vi "Generate Patch Seq Img Core-retd.vi"(0 "tdms file ref":refnum<k34>, 1 "Channel to process":enum16{"Red", "Green"}(ring), 5 "All header parameters":T1={"Imaging Protocol"=enum."AOL Z-Stack", "Number of POI"=0, "Number of Miniscans"=0, "Number of Trials"=0, "Number of Cycles "=0, "# Averaged Frames"=0, "Laser power (%)"=0, "Pockels"=0.0, "Acquisition Length (sec)"=0.0, "Fill time (us)"=0.0, "POI Dwell time (us)"=0.0, "Miniscan Dwell time per pixel (us)"=0.0, "PMT 1"=0.0, "PMT 2"=0.0, "Back Apperture"=0.0, "Zoom"=0.0, "Frame Size"=200, "Center Frequency"=0.0, "Field of View"=0.0, "DwellTime (us)"=0.0, "Wavelength (nm)"=0.0, "AOL Z"=0.0, "AOL Mode"=enum."Raster", "GridXY"=0.0, "GridZ"=0.0, "TriggerDelay (sec)"=0.0, "Number of Pixels in Miniscan"=0, "Experiment folder path"=path "", "X centre"=0.0, "Y centre"=0.0, "Angle (degrees)"=0.0, "Plane Mode"=0, "Software version"=0.0, "Objective"="Olympus  20X", "MotorZ Calibration"=0, "Pockels Calibration"=0, "Threshold"=[], "Video length (sec)"=0.0, "Frame rate (fps)"=0, "Rectangle ROI length (pixels)"=0, "Rectangle ROI height (pixels)"=0} {"Pockels" format="%#.6g"; "Software version" format="%#.6g"; "Plane Mode" items=["XY Plane", "XZ Plane", "YZ Plane", "arbitraryplane"]; "Angle (degrees)" format="%#.6g"; "Frame Size" items=["100X100"=100, "128X128"=128, "200X200"=200, "256X256"=256, "512X512"=512, "1024x1024"=1024, "2048x2048"=2048]; "Back Apperture" format="%#.6g"; "PMT 2" format="%#.6g"; "PMT 1" format="%#.6g"; "Miniscan Dwell time per pixel (us)" format="%#.6g"; "Zoom" format="%#.6g"; "POI Dwell time (us)" format="%#.6g"; "Acquisition Length (sec)" format="%#.6g"; "Fill time (us)" format="%#.6g"}, 7 "TDMS file path & name":path=path "C:/Users/Theo/Desktop/Datasets/140401_17_44_08-rig 3 debugging/Functional imaging TDMS data files/001.tdms", 9 "Patch Image Folder":path[](array[path]), 11 "error in (no error)":errorcluster, 13 "TIFF file handles":i32[](array[numeric]), 14 "Trial Number":i32) -> (4 "tdms file out":refnum<k34>, 15 "error out":errorcluster)   [LabVIEW 2020]
uses:
  User Interface/Visualisation/Functional Imaging Viewer/SubVIs/Experiment header interface/Typedefs/Header parameters cluster-ALL-retd.ctl
  Typedefs/Imaging Protocols enum.ctl
  Typedefs/Frame Size.ctl
  Typedefs/AOL modes.ctl
  Typedefs/Plane Mode.ctl
  Typedefs/Objective selector control enum.ctl
  Typedefs/Channel Selector.ctl
  Globals/gl_funct TIFF export globals.vi
  <vilib>/vision/NI_Vision_Development_Module.lvlib
panel:
  out "Loop time (ms)":u32
  # "Re-entrant"
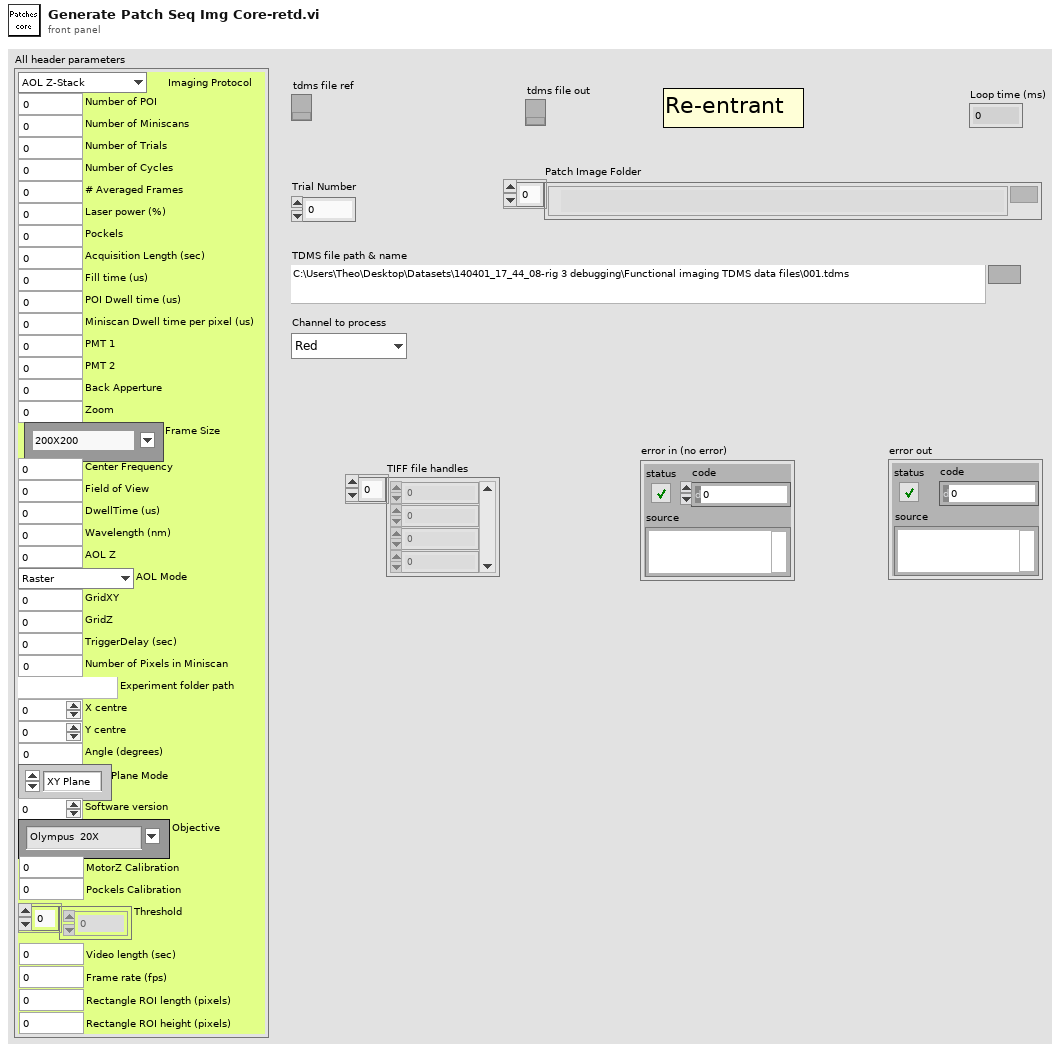
[diagram p1: front panel]
types:
  T1 = typedef "Header parameters cluster-ALL-retd.ctl" = cluster{"Imaging Protocol":T2, "Number of POI":u16, "Number of Miniscans":u16, "Number of Trials":u16, "Number of Cycles ":u64, "# Averaged Frames":u16, "Laser power (%)":u8, "Pockels":dbl, "Acquisition Length (sec)":dbl, "Fill time (us)":dbl, "POI Dwell time (us)":dbl, "Miniscan Dwell time per pixel (us)":dbl, "PMT 1":dbl, "PMT 2":dbl, "Back Apperture":dbl, "Zoom":dbl, "Frame Size":T3, "Center Frequency":dbl, "Field of View":dbl, "DwellTime (us)":dbl, "Wavelength (nm)":dbl, "AOL Z":dbl, "AOL Mode":T4, "GridXY":dbl, "GridZ":dbl, "TriggerDelay (sec)":dbl, "Number of Pixels in Miniscan":u16, "Experiment folder path":path, "X centre":dbl, "Y centre":dbl, "Angle (degrees)":dbl, "Plane Mode":T5, "Software version":dbl, "Objective":T6, "MotorZ Calibration":u32, "Pockels Calibration":u32, "Threshold":u16[], "Video length (sec)":dbl, "Frame rate (fps)":u8, "Rectangle ROI length (pixels)":u16, "Rectangle ROI height (pixels)":u16}
  T2 = typedef "Imaging Protocols enum.ctl" = enum16{"AOL Z-Stack", "Motor Z Stack", "Functional Acquisition", "Single Plane Acquisition", "Volume Acquisition", "Live Imaging", "Live Plane Imaging", "Live Volume Imaging"}
  T3 = typedef "Frame Size.ctl" = u16
  T4 = typedef "AOL modes.ctl" = enum16{"Raster", "Structural", "Pointing", "Mini Scan", "Alignment"}
  T5 = typedef "Plane Mode.ctl" = u16
  T6 = typedef "Objective selector control enum.ctl" = string
  T7 = typedef "Funct TIFF exporter ctrl refs.ctl" = cluster{"This VI":refnum<vi>, "Current Experiment":refnum<vi>, "Imaging protocol":refnum<vi>, "Predominant ROI type":refnum<vi>, "Patches in Experiment":refnum<vi>, "Folder Path":refnum<vi>, "Export":refnum<vi>, "Trial number":refnum<vi>, "Output TIFF type":refnum<vi>}
  T8 = typedef "Exported TIFF type.ctl" = enum16{"One multi-page TIFF file for each rectangle", "Individual TIFF files"}
  T9 = typedef "Channel Selector.ctl" = enum16{"Red Channel", "Green Channel", "Blended"}
  T10 = cluster{"Number of cycles":i32, "number of planes":i32, "number of miniscans in a Plane":i32, "number of pixels in a miniscan":i32}
  T11 = typedef "Image Type" = u32
  T12 = typedef "IMAQ Image.ctl" = refnum<image>
  T13 = typedef "IMAQ AVI2 Refnum.ctl" = refnum<k20>
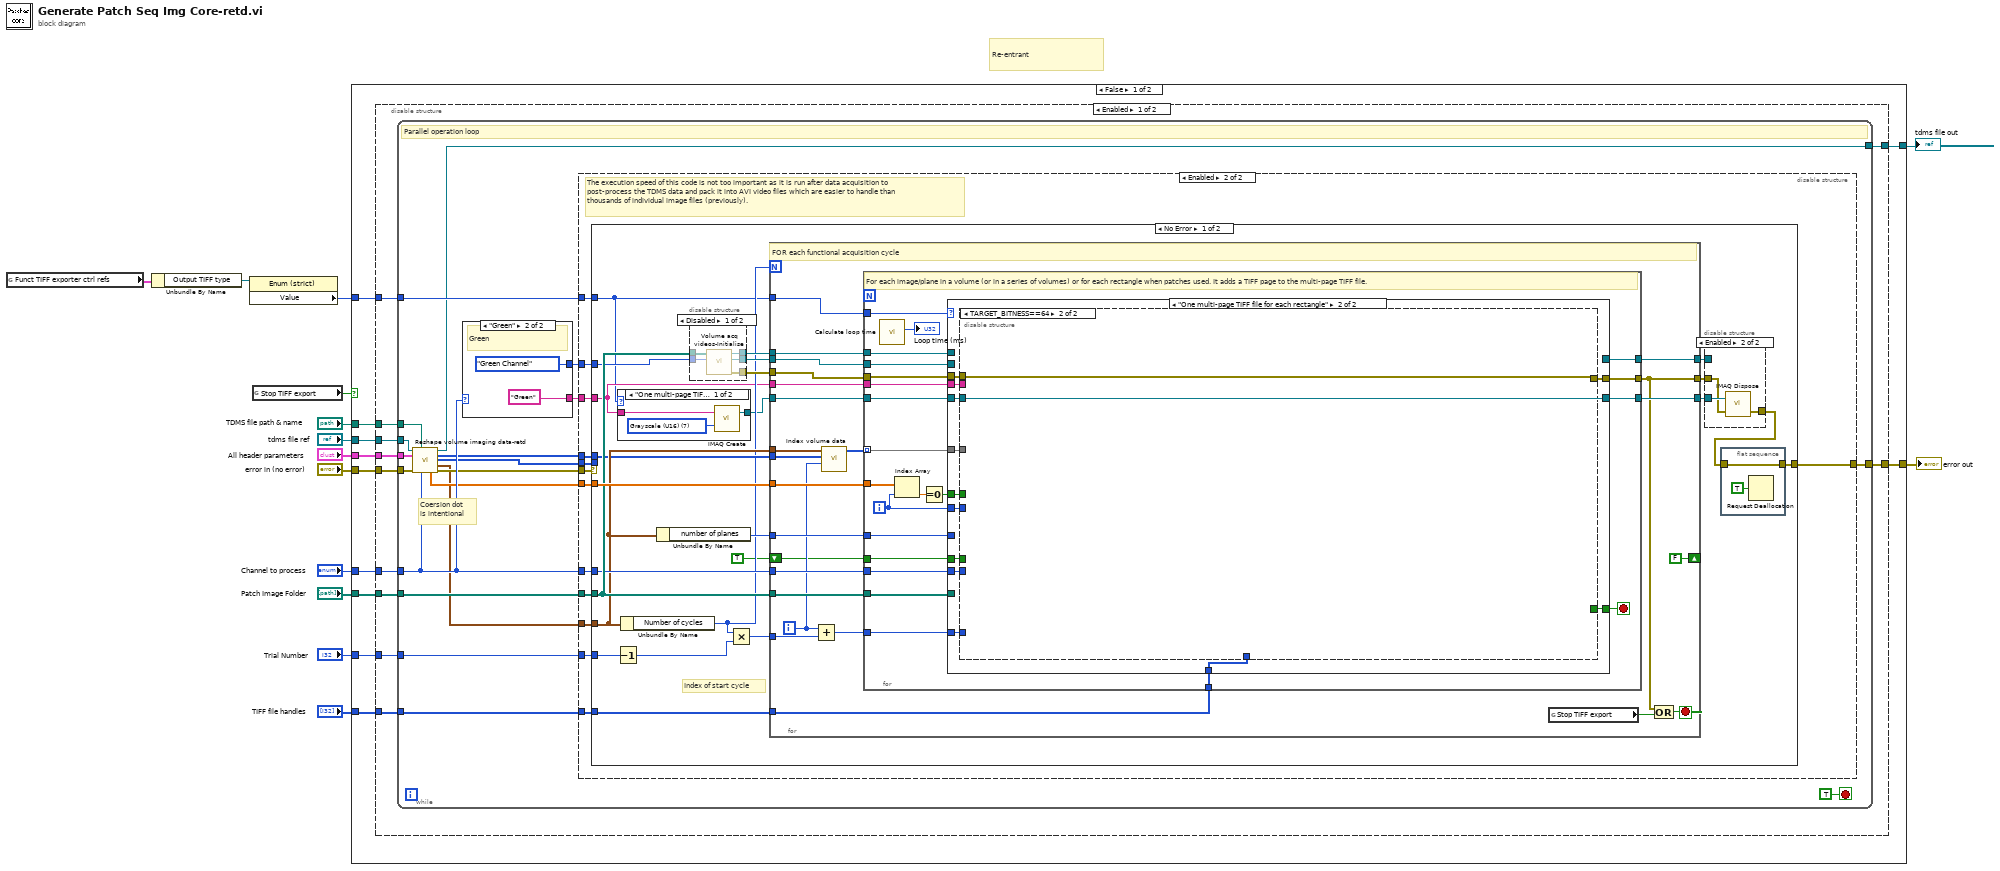
[diagram p0: block diagram]
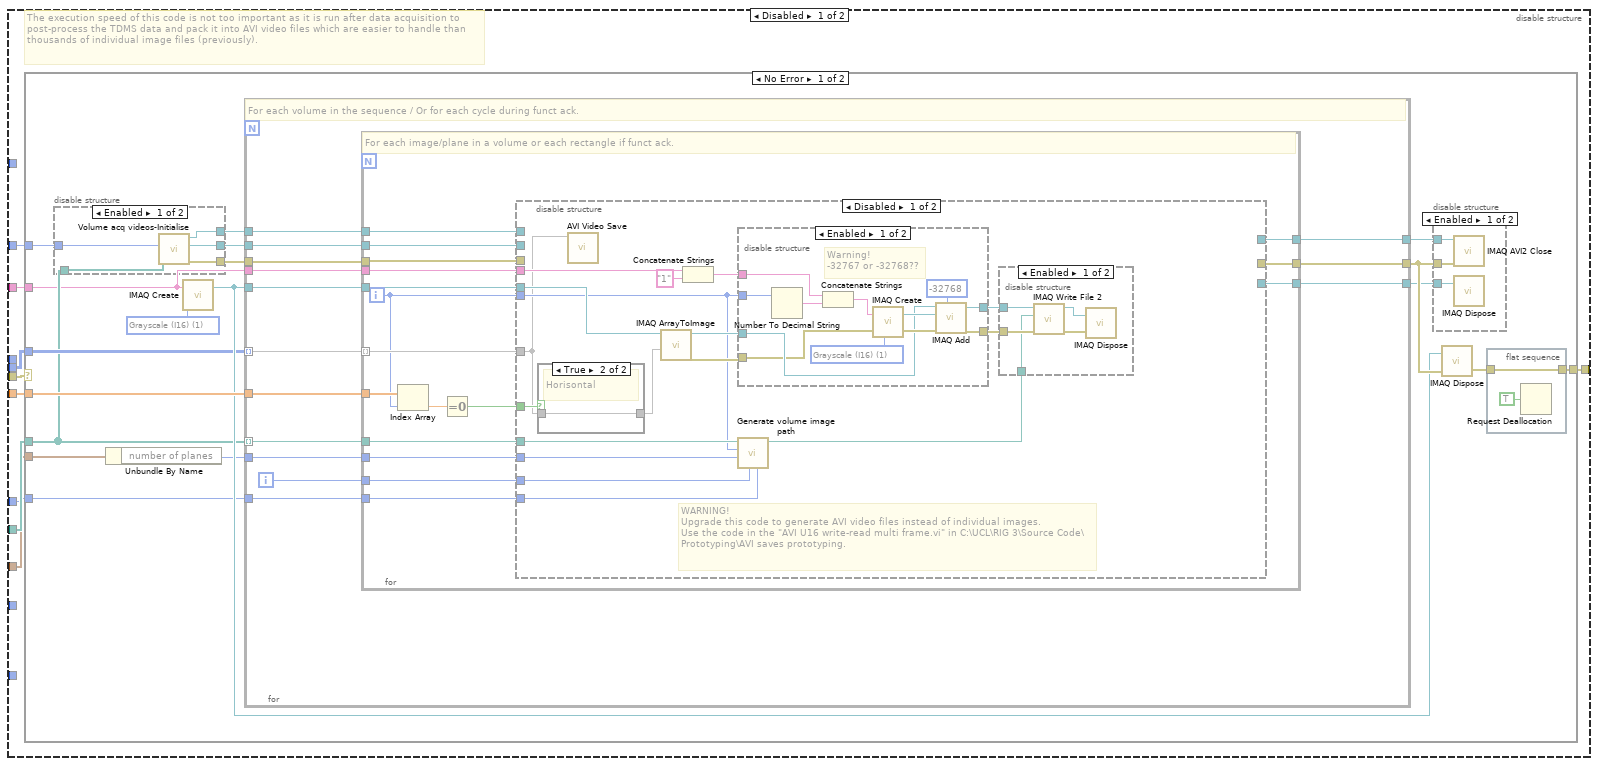
[diagram p2: hidden frame]
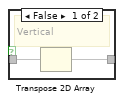
[diagram p5: hidden frame]
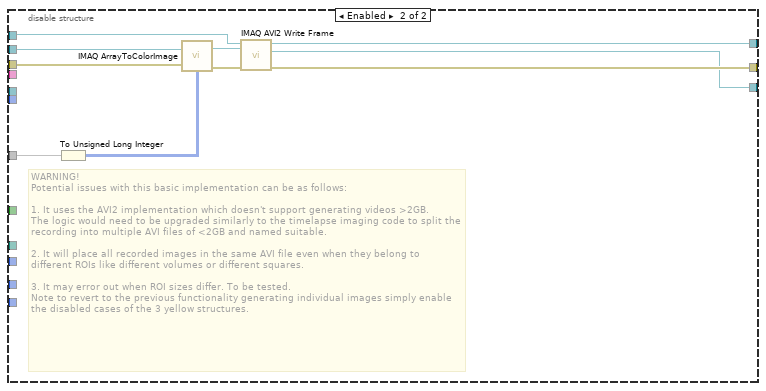
[diagram p8: hidden frame]
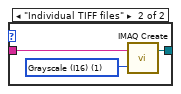
[diagram p10: hidden frame]
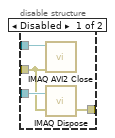
[diagram p12: hidden frame]
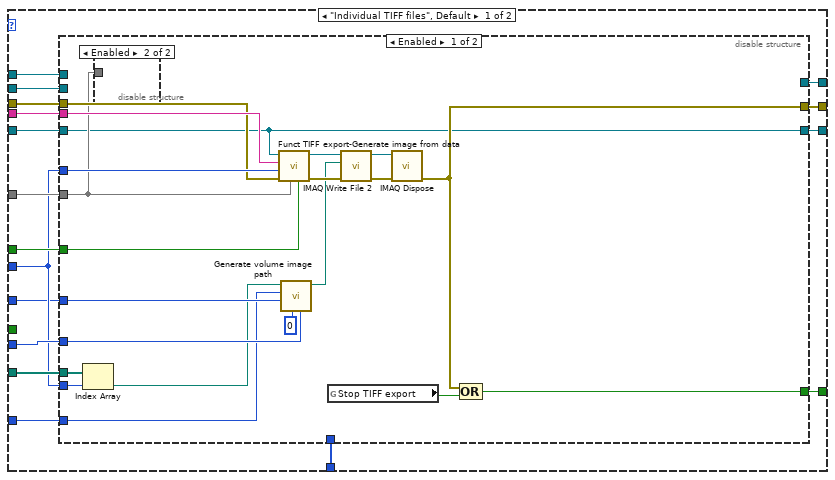
[diagram p13: hidden frame]
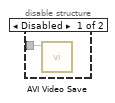
[diagram p14: hidden frame]
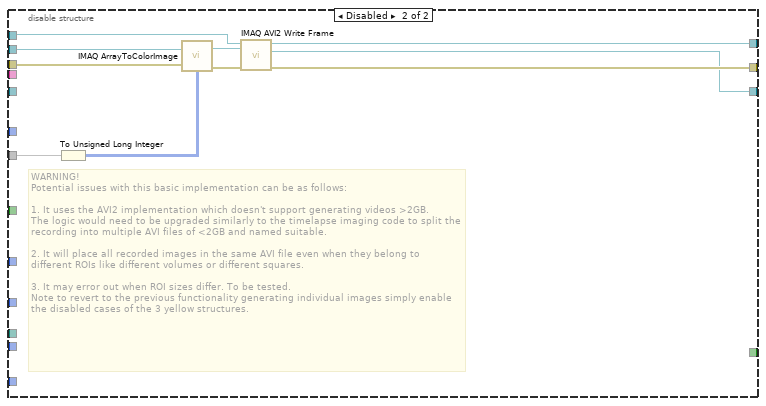
[diagram p15: hidden frame]
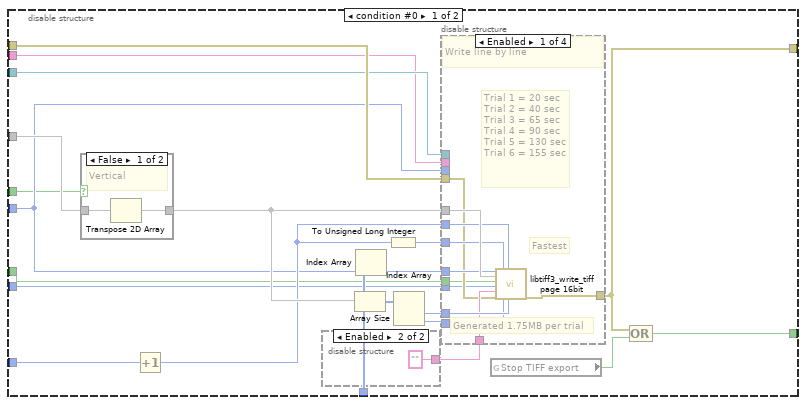
[diagram p16: hidden frame]
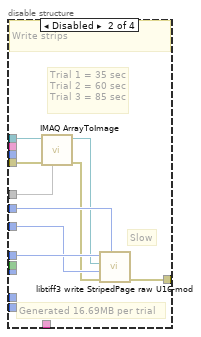
[diagram p17: hidden frame]
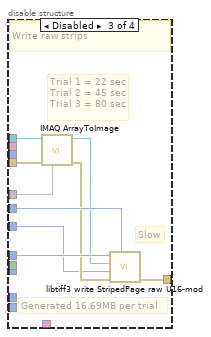
[diagram p18: hidden frame]
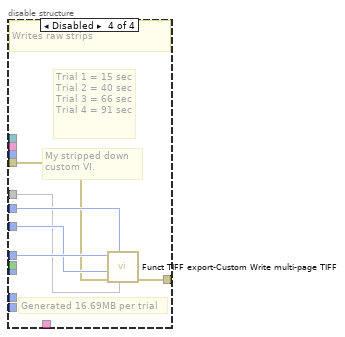
[diagram p19: hidden frame]
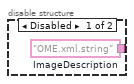
[diagram p20: hidden frame]
diagram:
  # "Re-entrant"
  n1 = global read "gl_funct TIFF export globals.vi" "Funct TIFF exporter ctrl refs"() -> (w6:T7)
  n2 = Unbundle By Name(w6) -> ("Output TIFF type"=w7:refnum<vi>)
  n3 = property on="Property Node" class="Enum (strict)"(reference=w7) -> ("Value"=w5:T8)  [unwired: 1 in, 2 out]
  n4 = global read "gl_funct TIFF export globals.vi" "Stop TIFF export"() -> (w10:bool)
  n5 = case shown="False" w10 {
    tunnel: [w25 w541] -> w14
    tunnel: "error in (no error)" -> [w24 w541]
    tunnel: "Channel to process" -> [w23 _]
    tunnel: "Patch Image Folder" -> [w22 _]
    tunnel: "Trial Number" -> [w21 _]
    tunnel: "TIFF file handles" -> [w20 _]
    tunnel: w5 -> [w19 _]
    tunnel: "tdms file ref" -> [w18 w540]
    tunnel: "All header parameters" -> [w17 _]
    tunnel: "TDMS file path & name" -> [w16 _]
    tunnel: [w15 w540] -> w1
    frame False {
      n6 = disable-structure shown="Enabled" {
        disable-tunnel: [w36 w412] -> w25
        disable-tunnel: w22 -> [w35 w411]
        disable-tunnel: w24 -> [w34 w410]
        disable-tunnel: w23 -> [w33 w409]
        disable-tunnel: w21 -> [w32 _]
        disable-tunnel: w20 -> [w31 _]
        disable-tunnel: w19 -> [w30 _]
        disable-tunnel: w18 -> [w29 w407]
        disable-tunnel: w17 -> [w28 w406]
        disable-tunnel: w16 -> [w27 w408]
        disable-tunnel: [w26 w405] -> w15
        frame Enabled {
          n7 = while {
            tunnel: [w55] -> w36
            tunnel: w35 -> [w54]
            tunnel: w34 -> [w53]
            tunnel: w33 -> [w52]
            tunnel: w32 -> [w51]
            tunnel: w31 -> [w50]
            tunnel: w30 -> [w49]
            tunnel: w29 -> [w38]
            tunnel: w28 -> [w41]
            tunnel: w27 -> [w40]
            tunnel: [w39] -> w26
            stop <- TRUE stop-if-true
            # "Coersion dot\nis intentional"
            # "Parallel operation loop"
            n8 = call "Reshape volume imaging data-retd.vi"("tdms file ref"=w38, "TDMS file path & name"=w40, "All header parameters"=w41, "error in (no error)"=w53, "Channel to process"=w52) -> ("tdms file out"=w39:refnum<k34>, "Single channel data"=w43:u16[], "Channel 4D data"=w42:u16[][][][], "Volumetric parameters"=w44:T10, "Angles (deg)"=w45:dbl[], "error out"=w47:errorcluster)  [unwired: 5 in]
            n9 = case shown="\"Green\"" w52 {
              tunnel: ["Red" ("Image Name") "Green" ("Image Name")] -> w48
              tunnel: [Channel_Selector."Red Channel" ("Channel") Channel_Selector."Green Channel" ("Channel")] -> w46
              frame "Red", Default {
                # "Red"
              }
              frame "Green" {
                # "Green"
              }
            }
            n10 = disable-structure shown="Enabled" {
              disable-tunnel: [w64 w186] -> w55
              disable-tunnel: w54 -> [w63 w185]
              disable-tunnel: w48 -> [w62 w184]
              disable-tunnel: w42 -> [w61 w183]
              disable-tunnel: w47 -> [w60 w182]
              disable-tunnel: w46 -> [w59 w181]
              disable-tunnel: w45 -> [w58 w180]
              disable-tunnel: w52 -> [w57 w179]
              disable-tunnel: w44 -> [w56 w178]
              disable-tunnel: w43 -> [_ w177]
              disable-tunnel: w51 -> [_ w175]
              disable-tunnel: w50 -> [_ w176]
              disable-tunnel: w49 -> [_ w174]
              frame Disabled {
                # "The execution speed of this code is not too important as it is run after data acquisition to post-process the TDMS data and pack it into AVI video files which are easier to handle than thousands of individual image files (previously)."
                n11 = case shown="No Error" w60 {
                  selector: w60 -> [_ w173]
                  tunnel: [w68 w173] -> w64
                  tunnel: w58 -> [w82 _]
                  tunnel: w61 -> [w74 _]
                  tunnel: w56 -> [w65 _]
                  tunnel: w63 -> [w71 _]
                  tunnel: w62 -> [w70 _]
                  tunnel: w57 -> [w67 _]
                  tunnel: w59 -> [w66 _]
                  frame No Error {
                    w73 = T11 1 items=["Grayscale (U8)", "Grayscale (I16)", "Grayscale (SGL)", "Complex (CSG)", "RGB (U32)", "HSL (U32)", "RGB (U64)", "Grayscale (U16)"] ("Image Type")
                    n12 = disable-structure "Diagram Disable Structure" shown="Enabled" {
                      disable-tunnel: [w89 _] -> w75
                      disable-tunnel: [w88 _] -> w76
                      disable-tunnel: [w87 _] -> w77
                      disable-tunnel: w71 -> [w86 _]
                      disable-tunnel: w66 -> [w85 _]
                      frame Enabled {
                        n13 = call "Volume acq videos-Initialise.vi"("Channel"=w85, "created path"=w86) -> ("error out"=w89:errorcluster, "Temp Image"=w88:T12, "Refnum out"=w87:T13)  [unwired: 7 in]
                      }
                      frame Disabled {
                      }
                    }
                    n14 = Unbundle By Name(w65) -> ("number of planes"=w72:i32)
                    n15 = call "IMAQ Create"("Image Name"=w70, "Image Type"=w73) -> ("New Image"=w80:T12)  [unwired: 3 in, 1 out]
                    n16 = for {
                      tunnel: w74 -> [w106] mode=indexing
                      tunnel: w80 -> [w105]
                      tunnel: w71 -> [w104] mode=indexing
                      tunnel: w72 -> [w102]
                      tunnel: w76 -> [w101]
                      tunnel: w77 -> [w100]
                      tunnel: w75 -> [w99]
                      tunnel: [w98] -> w81
                      tunnel: [w97] -> w78
                      tunnel: [w96] -> w79
                      tunnel: w82 -> [w95]
                      tunnel: w70 -> [w94]
                      tunnel: w67 -> [w93]
                      i -> [w103]
                      # "For each volume in the sequence / Or for each cycle during funct ack."
                      n17 = for {
                        tunnel: w106 -> [w110] mode=indexing
                        tunnel: w105 -> [w123]
                        tunnel: w104 -> [w122]
                        tunnel: w103 -> [w121]
                        tunnel: w102 -> [w120]
                        tunnel: w101 -> [w118]
                        tunnel: w100 -> [w119]
                        tunnel: w99 -> [w117]
                        tunnel: [w116] -> w98
                        tunnel: [w115] -> w97
                        tunnel: [w114] -> w96
                        tunnel: w95 -> [w109]
                        tunnel: w94 -> [w112]
                        tunnel: w93 -> [w111]
                        i -> [w108]
                        # "For each image/plane in a volume or each rectangle if funct ack."
                        n18 = Index Array(array=w109, index=w108) -> (element=w107:dbl)
                        n19 = Equal To 0?(x=w107) -> (x = 0?=w113:bool)
                        n20 = disable-structure shown="Disabled" {
                          disable-tunnel: w123 -> [w140 _]
                          disable-tunnel: w122 -> [w135 _]
                          disable-tunnel: w121 -> [w133 _]
                          disable-tunnel: w120 -> [w132 _]
                          disable-tunnel: w108 -> [w131 _]
                          disable-tunnel: w119 -> [_ w169]
                          disable-tunnel: w118 -> [_ w168]
                          disable-tunnel: w117 -> [_ w167]
                          disable-tunnel: [_ w166] -> w116
                          disable-tunnel: [_ w165] -> w115
                          disable-tunnel: [_ w164] -> w114
                          disable-tunnel: w113 -> [w130 _]
                          disable-tunnel: w110 -> [w125 w163]
                          disable-tunnel: w112 -> [w128 _]
                          disable-tunnel: w111 -> [w124 _]
                          frame Disabled {
                            # "WARNING!\nUpgrade this code to generate AVI video files instead of individual images.\nUse the code in the \"AVI U16 write-read multi frame.vi\" in C:\\UCL\\RIG 3\\Source Code\\Prototyping\\AVI saves prototyping."
                            n21 = case shown="True" w130 {
                              tunnel: w125 -> [w142 w143]
                              tunnel: [w141 w143] -> w129
                              frame False {
                                # "Vertical"
                                n22 = Transpose 2D Array(2D array=w142) -> (transposed array=w141:u16[][])
                              }
                              frame True {
                                # "Horisontal"
                              }
                            }
                            n23 = call "AVI Video Save.vi"("Image Pixels"=w125) -> ()  [unwired: 9 in, 2 out]
                            n24 = call "IMAQ ArrayToImage"("Image Pixels (I16)"=w129, "Image"=w140) -> ("error out"=w136:errorcluster, "Image Out"=w139:T12)  [unwired: 8 in]
                            n25 = Concatenate Strings(w128, "1" ("string")) -> (w126:string)
                            n26 = call "Generate volume image path.vi"("Channel to process"=w124, "Volume index"=w133, "Number of planes"=w132, "Plane index (within its volume)"=w131, "Folder path"=w135) -> ("File path"=w134:path)  [unwired: 5 in, 1 out]
                            n27 = disable-structure shown="Enabled" {
                              disable-tunnel: w131 -> [w154 _]
                              disable-tunnel: w139 -> [w153 w162]
                              disable-tunnel: [w152 w162] -> w138
                              disable-tunnel: [w150 w161] -> w137
                              disable-tunnel: w136 -> [w151 w161]
                              disable-tunnel: w126 -> [w149 _]
                              frame Enabled {
                                w156 = T11 1 items=["Grayscale (U8)", "Grayscale (I16)", "Grayscale (SGL)", "Complex (CSG)", "RGB (U32)", "HSL (U32)", "RGB (U64)"] ("Image Type")
                                # "Warning!\n-32767 or -32768??"
                                n28 = Number To Decimal String(number=w154) -> (decimal integer string=w157:string)  [unwired: 1 in]
                                n29 = Concatenate Strings(w149, w157) -> (w158:string)
                                n30 = call "IMAQ Create"("Image Name"=w158, "Image Type"=w156, "error in (no error)"=w151) -> ("New Image"=w159:T12, "error out"=w160:errorcluster)  [unwired: 2 in]
                                n31 = call "IMAQ Add"("Image Src A"=w153, "Constant"=i16 -32768, "Image Dst"=w159, "error in (no error)"=w160) -> ("Image Dst Out"=w152:T12, "error out"=w150:errorcluster)  [unwired: 3 in]
                              }
                              frame Disabled {
                              }
                            }
                            n32 = disable-structure shown="Enabled" {
                              disable-tunnel: w138 -> [w146 _]
                              disable-tunnel: w137 -> [w145 _]
                              disable-tunnel: w134 -> [w144 _]
                              frame Enabled {
                                n33 = call-poly "IMAQ Write File 2"("error in (no error)"=w145, "File Path"=w144, "Image"=w146) -> ("error out"=w148:errorcluster, "Image Out (duplicate)"=w147:T12)  [unwired: 7 in]
                                n34 = call "IMAQ Dispose"("Image"=w147, "error in (no error)"=w148) -> ()  [unwired: 4 in, 1 out]
                              }
                              frame Disabled {
                              }
                            }
                          }
                          frame Enabled {
                            # "WARNING!\nPotential issues with this basic implementation can be as follows:\n\n1. It uses the AVI2 implementation which doesn't support generating videos >2GB. \nThe logic would need to be upgraded similarly to the timelapse imaging code to split the recording into multiple AVI files of <2GB and named suitable.\n\n2. It will place all recorded images in the same AVI file even when they belong to different ROIs like different volumes or different squares.\n\n3. It may error out when ROI sizes differ. To be tested.\nNote to revert to the previous functionality generating individual images simply enable the disabled cases of the 3 yellow structures."
                            n35 = To Unsigned Long Integer(number=w163) -> (unsigned 32bit integer=w171:u32[][])
                            n36 = call "IMAQ ArrayToColorImage"("Image Pixels (U32)"=w171, "Image"=w168, "error in (no error)"=w167) -> ("Image Out"=w172:T12, "error out"=w170:errorcluster)  [unwired: 1 in, 1 out]
                            n37 = call "IMAQ AVI2 Write Frame"("error in (no error)"=w170, "Image"=w172, "AVI Refnum"=w169) -> ("error out"=w166:errorcluster, "Image Out (duplicate)"=w164:T12, "AVI Refnum (duplicate)"=w165:T13)  [unwired: 6 in]
                          }
                        }
                      }
                    }
                    n38 = disable-structure "Diagram Disable Structure" shown="Enabled" {
                      disable-tunnel: w78 -> [w92 _]
                      disable-tunnel: w81 -> [w91 _]
                      disable-tunnel: w79 -> [w90 _]
                      frame Enabled {
                        n39 = call "IMAQ AVI2 Close"("error in (no error)"=w91, "AVI Refnum"=w92) -> ()  [unwired: 9 in, 1 out]
                        n40 = call "IMAQ Dispose"("Image"=w90) -> ()  [unwired: 5 in, 1 out]
                      }
                      frame Disabled {
                      }
                    }
                    n41 = call "IMAQ Dispose"("Image"=w80, "error in (no error)"=w81) -> ("error out"=w69:errorcluster)  [unwired: 4 in]
                    n42 = flat-sequence {
                      tunnel: w69 -> [w83]
                      tunnel: [w83] -> w68
                      frame #0 {
                        n43 = Request Deallocation(TRUE ("flag")) -> ()
                      }
                    }
                  }
                  frame Error {
                  }
                }
              }
              frame Enabled {
                # "The execution speed of this code is not too important as it is run after data acquisition to post-process the TDMS data and pack it into AVI video files which are easier to handle than thousands of individual image files (previously)."
                n44 = case shown="No Error" w182 {
                  selector: w182 -> [_ w400]
                  tunnel: [w202 w400] -> w186
                  tunnel: w180 -> [w210 _]
                  tunnel: w183 -> [_ _]
                  tunnel: w178 -> [w199 _]
                  tunnel: w185 -> [w203 _]
                  tunnel: w184 -> [w190 _]
                  tunnel: w179 -> [w201 _]
                  tunnel: w181 -> [w200 _]
                  tunnel: w177 -> [w198 _]
                  tunnel: w175 -> [w196 _]
                  tunnel: w176 -> [w195 _]
                  tunnel: w174 -> [w188 _]
                  frame No Error {
                    # "Index of start cycle"
                    n45 = Decrement(x=w196) -> (x-1=w194:i32)
                    n46 = case shown="\"One multi-page TIFF file for each rectangle\"" w188 {
                      tunnel: w190 -> [w212 w215]
                      tunnel: [w211 w214] -> w189
                      frame "One multi-page TIFF file for each rectangle" {
                        w213 = T11 7 items=["Grayscale (U8)", "Grayscale (I16)", "Grayscale (SGL)", "Complex (CSG)", "RGB (U32)", "HSL (U32)", "RGB (U64)", "Grayscale (U16)"] ("Image Type")
                        n47 = call "IMAQ Create"("Image Name"=w212, "Image Type"=w213) -> ("New Image"=w211:T12)  [unwired: 3 in, 1 out]
                      }
                      frame "Individual TIFF files" {
                        w216 = T11 1 items=["Grayscale (U8)", "Grayscale (I16)", "Grayscale (SGL)", "Complex (CSG)", "RGB (U32)", "HSL (U32)", "RGB (U64)", "Grayscale (U16)"] ("Image Type")
                        n48 = call "IMAQ Create"("Image Name"=w215, "Image Type"=w216) -> ("New Image"=w214:T12)  [unwired: 3 in, 1 out]
                      }
                    }
                    n49 = Unbundle By Name(w199) -> ("Number of cycles"=w191:i32)
                    n50 = Unbundle By Name(w199) -> ("number of planes"=w204:i32)
                    n51 = disable-structure shown="Disabled" {
                      disable-tunnel: [w221 _] -> w207
                      disable-tunnel: [w220 _] -> w206
                      disable-tunnel: [w219 _] -> w205
                      disable-tunnel: w203 -> [w218 _]
                      disable-tunnel: w200 -> [w217 _]
                      frame Disabled {
                        n52 = call "Volume acq videos-Initialise.vi"("Channel"=w217, "created path"=w218) -> ("error out"=w219:errorcluster, "Temp Image"=w220:T12, "Refnum out"=w221:T13)  [unwired: 7 in]
                      }
                      frame Enabled {
                      }
                    }
                    n53 = Multiply(x=w191, y=w194) -> (x*y=w197:i32)
                    n54 = for {
                      N: w191 -> [_]
                      tunnel: w189 -> [w254]
                      tunnel: w203 -> [w253]
                      tunnel: w204 -> [w252]
                      tunnel: w206 -> [w251]
                      tunnel: w207 -> [w250]
                      tunnel: w205 -> [w249]
                      tunnel: [w233] -> w193
                      tunnel: [w248] -> w208
                      tunnel: [w247] -> w209
                      tunnel: w210 -> [w246]
                      tunnel: w190 -> [w245]
                      tunnel: w201 -> [w244]
                      tunnel: w199 -> [w242]
                      tunnel: w198 -> [w241]
                      tunnel: w197 -> [w238]
                      tunnel: w195 -> [w237]
                      tunnel: w188 -> [w234]
                      shift-right: [FALSE] -> _
                      shift-left: TRUE -> [w232]
                      i -> [w239]
                      stop <- w236 stop-if-true
                      # "FOR each functional acquisition cycle"
                      n55 = Add(x=w239, y=w238) -> (x+y=w240:i32)
                      n56 = call "Index volume data.vi"("Cycle index"=w239, "Single trial data (single channel)"=w241, "Parameters Cluster"=w242) -> ("3D"=w243:u16[][][])  [unwired: 5 in, 3 out]
                      n57 = for {
                        tunnel: w243 -> [w256] mode=indexing
                        tunnel: w254 -> [w276]
                        tunnel: w253 -> [w275]
                        tunnel: w252 -> [w261]
                        tunnel: w251 -> [w273]
                        tunnel: w250 -> [w274]
                        tunnel: w249 -> [w272]
                        tunnel: [w271] -> w233
                        tunnel: [w270] -> w248
                        tunnel: [w269] -> w247
                        tunnel: w246 -> [w265]
                        tunnel: w245 -> [w267]
                        tunnel: w244 -> [w266]
                        tunnel: w240 -> [w263]
                        tunnel: w237 -> [w259]
                        tunnel: w234 -> [w258]
                        tunnel: w232 -> [w255]
                        i -> [w262]
                        stop <- w260 stop-if-true
                        # "For each image/plane in a volume (or in a series of volumes) or for each rectangle when patches used. It adds a TIFF page to the multi-page TIFF file."
                        n58 = call <userlib>:"Calculate loop time.vi"() -> ("Loop time (ms)"=→"Loop time (ms)":u32)  [unwired: 11 in]
                        n59 = Index Array(array=w265, index=w262) -> (element=w264:dbl)
                        n60 = Equal To 0?(x=w264) -> (x = 0?=w268:bool)
                        n61 = case shown="\"One multi-page TIFF file for each rectangle\"" w258 {
                          tunnel: w276 -> [w293 w332]
                          tunnel: w275 -> [w292 _]
                          tunnel: w274 -> [w291 _]
                          tunnel: w273 -> [w290 _]
                          tunnel: w272 -> [w289 w333]
                          tunnel: [w288 w328] -> w271
                          tunnel: [w287 _] -> w270
                          tunnel: [w286 w332] -> w269
                          tunnel: w268 -> [w285 w329]
                          tunnel: w267 -> [w284 w331]
                          tunnel: w266 -> [w283 w327]
                          tunnel: w256 -> [w282 w334]
                          tunnel: w263 -> [w281 w335]
                          tunnel: w262 -> [w280 w330]
                          tunnel: w261 -> [w279 _]
                          tunnel: [w278 w337] -> w260
                          tunnel: w259 -> [w277 w336]
                          tunnel: w255 -> [_ w326]
                          frame "Individual TIFF files", Default {
                            n62 = disable-structure shown="Enabled" {
                              disable-tunnel: w293 -> [w294 _]
                              disable-tunnel: w292 -> [w307 _]
                              disable-tunnel: w279 -> [w312 _]
                              disable-tunnel: w280 -> [w311 _]
                              disable-tunnel: w291 -> [_ w322]
                              disable-tunnel: w290 -> [_ w321]
                              disable-tunnel: w289 -> [w297 w320]
                              disable-tunnel: [w303 w319] -> w288
                              disable-tunnel: [_ w318] -> w287
                              disable-tunnel: [w294 w317] -> w286
                              disable-tunnel: w285 -> [w296 _]
                              disable-tunnel: w282 -> [w295 w316]
                              disable-tunnel: w284 -> [w310 _]
                              disable-tunnel: w283 -> [w309 _]
                              disable-tunnel: w280 -> [w302 _]
                              disable-tunnel: w281 -> [w306 _]
                              disable-tunnel: [w304 _] -> w278
                              disable-tunnel: w277 -> [_ _]
                              frame Enabled {
                                n63 = Index Array(array=w307, index=w302) -> (element=w308:path)
                                n64 = disable-structure shown="Enabled" {
                                disable-tunnel: w295 -> [w315 _]
                                frame Disabled {
                                n65 = call "AVI Video Save.vi"("Image Pixels"=w315) -> ()  [unwired: 9 in, 2 out]
                                }
                                frame Enabled {
                                }
                                }
                                n66 = call "Funct TIFF export-Generate image from data.vi"("Horisontal (T)"=w296, "3D"=w295, "error in (no error)"=w297, "Rectangle index"=w311, "Image Name"=w310, "Refnum in"=w294) -> ("error out"=w313:errorcluster, "Refnum out"=w314:T12)  [unwired: 4 in]
                                n67 = call "Generate volume image path.vi"("Channel to process"=w309, "Volume index"=0, "Number of planes"=w312, "Plane index (within its volume)"=w306, "Folder path"=w308) -> ("File path"=w299:path)  [unwired: 5 in, 1 out]
                                n68 = global read "gl_funct TIFF export globals.vi" "Stop TIFF export"() -> (w305:bool)
                                n69 = call-poly "IMAQ Write File 2"("error in (no error)"=w313, "File Path"=w299, "Image"=w314) -> ("error out"=w301:errorcluster, "Image Out (duplicate)"=w300:T12)  [unwired: 7 in]
                                n70 = call "IMAQ Dispose"("Image"=w300, "error in (no error)"=w301) -> ("error out"=w303:errorcluster)  [unwired: 4 in]
                                n71 = Compound Arithmetic op=OR(w303, w305) -> (w304:bool)
                              }
                              frame Disabled {
                                # "WARNING!\nPotential issues with this basic implementation can be as follows:\n\n1. It uses the AVI2 implementation which doesn't support generating videos >2GB. \nThe logic would need to be upgraded similarly to the timelapse imaging code to split the recording into multiple AVI files of <2GB and named suitable.\n\n2. It will place all recorded images in the same AVI file even when they belong to different ROIs like different volumes or different squares.\n\n3. It may error out when ROI sizes differ. To be tested.\nNote to revert to the previous functionality generating individual images simply enable the disabled cases of the 3 yellow structures."
                                n72 = To Unsigned Long Integer(number=w316) -> (unsigned 32bit integer=w324:u32[][])
                                n73 = call "IMAQ ArrayToColorImage"("Image Pixels (U32)"=w324, "Image"=w321, "error in (no error)"=w320) -> ("Image Out"=w325:T12, "error out"=w323:errorcluster)  [unwired: 1 in, 1 out]
                                n74 = call "IMAQ AVI2 Write Frame"("error in (no error)"=w323, "Image"=w325, "AVI Refnum"=w322) -> ("error out"=w319:errorcluster, "Image Out (duplicate)"=w317:T12, "AVI Refnum (duplicate)"=w318:T13)  [unwired: 6 in]
                              }
                            }
                          }
                          frame "One multi-page TIFF file for each rectangle" {
                            n75 = disable-structure shown="TARGET_BITNESS==64" {
                              disable-tunnel: [w358 _] -> w337
                              disable-tunnel: w336 -> [w357 _]
                              disable-tunnel: w335 -> [w351 _]
                              disable-tunnel: w334 -> [w350 _]
                              disable-tunnel: w333 -> [w345 w399]
                              disable-tunnel: w332 -> [w344 _]
                              disable-tunnel: w331 -> [w343 _]
                              disable-tunnel: w330 -> [w342 _]
                              disable-tunnel: w329 -> [w341 _]
                              disable-tunnel: [w340 w399] -> w328
                              disable-tunnel: w327 -> [w339 _]
                              disable-tunnel: w326 -> [w338 _]
                              frame condition #0 {
                                n76 = case shown="False" w341 {
                                tunnel: w350 -> [w397 w398]
                                tunnel: [w396 w398] -> w356
                                frame False {
                                # "Vertical"
                                n77 = Transpose 2D Array(2D array=w397) -> (transposed array=w396:u16[][])
                                }
                                frame True {
                                # "Horisontal"
                                }
                                }
                                n78 = Increment(x=w351) -> (x+1=w348:i32)
                                n79 = disable-structure shown="Enabled" {
                                disable-tunnel: [w394 "" ("ImageDescription")] -> w352
                                frame Disabled {
                                w394 = "OME.xml.string"  # ImageDescription
                                }
                                frame Enabled {
                                }
                                }
                                n80 = Array Size(array=w356) -> (size(s)=w355:i32[])
                                n81 = Index Array(array=w357, index=w342) -> (element=w349:i32)
                                n82 = To Unsigned Long Integer(number=w348) -> (unsigned 32bit integer=w347:u32)
                                n83 = Index Array(array=w355) -> (element #1=w354:i32, element #2=w353:i32)  [unwired: 2 in]
                                n84 = disable-structure shown="Enabled" {
                                disable-tunnel: [w369 w371 w382 w390] -> w340
                                disable-tunnel: w356 -> [w368 w372 w385 w389]
                                disable-tunnel: w354 -> [w367 _ _ _]
                                disable-tunnel: w353 -> [w366 _ _ _]
                                disable-tunnel: w352 -> [w365 _ _ _]
                                disable-tunnel: w349 -> [w364 w377 w383 w392]
                                disable-tunnel: w348 -> [w363 w378 w384 w393]
                                disable-tunnel: w347 -> [w362 w376 w379 w391]
                                disable-tunnel: w345 -> [w361 w373 w386 w388]
                                disable-tunnel: w344 -> [_ w375 w387 _]
                                disable-tunnel: w343 -> [_ _ _ _]
                                disable-tunnel: w342 -> [_ _ _ _]
                                disable-tunnel: w339 -> [w360 _ _ _]
                                disable-tunnel: w338 -> [w359 _ _ _]
                                frame Enabled {
                                # "Trial 1 = 20 sec\nTrial 2 = 40 sec\nTrial 3 = 65 sec\nTrial 4 = 90 sec\nTrial 5 = 130 sec\nTrial 6 = 155 sec"
                                # "Fastest"
                                # "Generated 1.75MB per trial"
                                # "Write line by line"
                                n85 = call "libtiff3_write_tiff page 16bit.vi"("Handle"=w364, "Image Pixels (U16)"=w368, "Reset"=w359, "Channel to process"=w360, "ImageDescription"=w365, "error in (no error)"=w361, "page"=w362, "x.pixels"=w366, "totalpages"=w363, "y.pixels"=w367) -> ("error out"=w369:errorcluster)  [unwired: 8 in, 1 out]
                                }
                                frame Disabled {
                                # "Trial 1 = 35 sec\nTrial 2 = 60 sec\nTrial 3 = 85 sec"
                                # "Slow"
                                # "Generated 16.69MB per trial"
                                # "Write strips"
                                n86 = call "IMAQ ArrayToImage"("Image Pixels (U16)"=w372, "error in (no error)"=w373, "Image"=w375) -> ("error out"=w374:errorcluster, "Image Out"=w370:T12)  [unwired: 7 in]
                                n87 = call "libtiff3 write StripedPage raw U16-mod.vi"("totalpages"=w378, "error in (no error)"=w374, "page"=w376, "Image"=w370, "Handle"=w377) -> ("error out"=w371:errorcluster)  [unwired: 5 in, 1 out]
                                }
                                frame Disabled {
                                # "Slow"
                                # "Trial 1 = 22 sec\nTrial 2 = 45 sec\nTrial 3 = 80 sec"
                                # "Generated 16.69MB per trial"
                                # "Write raw strips"
                                n88 = call "IMAQ ArrayToImage"("Image Pixels (U16)"=w385, "error in (no error)"=w386, "Image"=w387) -> ("error out"=w381:errorcluster, "Image Out"=w380:T12)  [unwired: 7 in]
                                n89 = call "libtiff3 write StripedPage raw U16-mod.vi"("totalpages"=w384, "error in (no error)"=w381, "page"=w379, "Image"=w380, "Handle"=w383) -> ("error out"=w382:errorcluster)  [unwired: 5 in, 1 out]
                                }
                                frame Disabled {
                                # "My stripped down\ncustom VI."
                                # "Trial 1 = 15 sec\nTrial 2 = 40 sec\nTrial 3 = 66 sec\nTrial 4 = 91 sec"
                                # "Generated 16.69MB per trial"
                                # "Writes raw strips"
                                n90 = call "Funct TIFF export-Custom Write multi-page TIFF.vi"("Image Pixels (U16)"=w389, "totalpages"=w393, "error in (no error)"=w388, "page"=w391, "Handle"=w392) -> ("error out"=w390:errorcluster)  [unwired: 5 in, 1 out]
                                }
                                }
                                n91 = global read "gl_funct TIFF export globals.vi" "Stop TIFF export"() -> (w346:bool)
                                n92 = Compound Arithmetic op=OR(w340, w346) -> (w358:bool)
                              }
                              frame condition #1 (active) {
                              }
                            }
                          }
                        }
                      }
                      n93 = global read "gl_funct TIFF export globals.vi" "Stop TIFF export"() -> (w235:bool)
                      n94 = Compound Arithmetic op=OR(w233, w235) -> (w236:bool)
                    }
                    n95 = disable-structure "Diagram Disable Structure" shown="Enabled" {
                      disable-tunnel: w208 -> [w227 _]
                      disable-tunnel: w193 -> [w224 w229]
                      disable-tunnel: w209 -> [w226 w230]
                      disable-tunnel: [w225 w228] -> w192
                      frame Disabled {
                        n96 = call "IMAQ AVI2 Close"("error in (no error)"=w224, "AVI Refnum"=w227) -> ()  [unwired: 9 in, 1 out]
                        n97 = call "IMAQ Dispose"("Image"=w226, "error in (no error)"=w224) -> ("error out"=w225:errorcluster)  [unwired: 4 in]
                      }
                      frame Enabled {
                        n98 = call "IMAQ Dispose"("Image"=w230, "error in (no error)"=w229) -> ("error out"=w228:errorcluster)  [unwired: 4 in]
                      }
                    }
                    n99 = flat-sequence {
                      tunnel: w192 -> [w222]
                      tunnel: [w222] -> w202
                      frame #0 {
                        n100 = Request Deallocation(TRUE ("flag")) -> ()
                      }
                    }
                  }
                  frame Error {
                  }
                }
              }
            }
          }
        }
        frame Disabled {
          # "The While Loop causes all instances of this VI to execute in parallel. (While loop is REDUNDANT)"
          n101 = while {
            tunnel: [w426] -> w412
            tunnel: w411 -> [w425]
            tunnel: w408 -> [w415]
            tunnel: w410 -> [w422]
            tunnel: w406 -> [w419]
            tunnel: w409 -> [w416]
            tunnel: w407 -> [w414]
            tunnel: [w413] -> w405
            stop <- TRUE stop-if-true
            # "The execution speed of this code is not too important as it is run after data acquisition to post-process the TDMS data and pack it into AVI video files which are easier to handle than thousands of individual image files (previously)."
            n102 = call "Reshape volume imaging data.vi"("tdms file ref"=w414, "TDMS file path & name"=w415, "All header parameters"=w419, "error in (no error)"=w422, "Channel to process"=w416) -> ("tdms file out"=w413:refnum<k34>, "Volumetric parameters"=w417:T10, "Angles (deg)"=w418:dbl[], "error out"=w423:errorcluster)  [unwired: 5 in, 2 out]
            n103 = case shown="\"Green\"" w416 {
              tunnel: ["Red" ("Image Name") "Green" ("Image Name")] -> w424
              tunnel: [Channel_Selector."Red Channel" ("Channel") Channel_Selector."Green Channel" ("Channel")] -> w421
              frame "Red", Default {
                # "Red"
              }
              frame "Green" {
                # "Green"
              }
            }
            n104 = case shown="No Error" w423 {
              selector: w423 -> [_ w539]
              tunnel: [w433 w539] -> w426
              tunnel: w418 -> [w448 _]
              tunnel: w413 -> [w440 _]
              tunnel: w417 -> [w437 _]
              tunnel: w425 -> [w436 _]
              tunnel: w424 -> [w435 _]
              tunnel: w416 -> [w432 _]
              tunnel: w421 -> [w431 _]
              frame No Error {
                w439 = T11 1 items=["Grayscale (U8)", "Grayscale (I16)", "Grayscale (SGL)", "Complex (CSG)", "RGB (U32)", "HSL (U32)", "RGB (U64)", "Grayscale (U16)"] ("Image Type")
                n105 = disable-structure "Diagram Disable Structure" shown="Enabled" {
                  disable-tunnel: [w455 _] -> w441
                  disable-tunnel: [w454 _] -> w442
                  disable-tunnel: [w453 _] -> w443
                  disable-tunnel: w436 -> [w452 _]
                  disable-tunnel: w431 -> [w451 _]
                  frame Enabled {
                    n106 = call "Volume acq videos-Initialise.vi"("Channel"=w451, "created path"=w452) -> ("error out"=w455:errorcluster, "Temp Image"=w454:T12, "Refnum out"=w453:T13)  [unwired: 7 in]
                  }
                  frame Disabled {
                  }
                }
                n107 = Unbundle By Name(w437) -> ("number of planes"=w438:i32)
                n108 = call "IMAQ Create"("Image Name"=w435, "Image Type"=w439) -> ("New Image"=w446:T12)  [unwired: 3 in, 1 out]
                n109 = for {
                  tunnel: w440 -> [w472]
                  tunnel: w446 -> [w471]
                  tunnel: w436 -> [w470] mode=indexing
                  tunnel: w438 -> [w468]
                  tunnel: w442 -> [w467]
                  tunnel: w443 -> [w466]
                  tunnel: w441 -> [w465]
                  tunnel: [w464] -> w447
                  tunnel: [w463] -> w444
                  tunnel: [w462] -> w445
                  tunnel: w448 -> [w461]
                  tunnel: w435 -> [w460]
                  tunnel: w432 -> [w459]
                  i -> [w469]
                  # "For each volume in the sequence / Or for each cycle during funct ack."
                  n110 = for {
                    tunnel: w472 -> [w476]
                    tunnel: w471 -> [w489]
                    tunnel: w470 -> [w488]
                    tunnel: w469 -> [w487]
                    tunnel: w468 -> [w486]
                    tunnel: w467 -> [w484]
                    tunnel: w466 -> [w485]
                    tunnel: w465 -> [w483]
                    tunnel: [w482] -> w464
                    tunnel: [w481] -> w463
                    tunnel: [w480] -> w462
                    tunnel: w461 -> [w475]
                    tunnel: w460 -> [w478]
                    tunnel: w459 -> [w477]
                    i -> [w474]
                    # "For each image/plane in a volume or each rectangle if funct ack."
                    n111 = Index Array(array=w475, index=w474) -> (element=w473:dbl)
                    n112 = Equal To 0?(x=w473) -> (x = 0?=w479:bool)
                    n113 = disable-structure shown="Disabled" {
                      disable-tunnel: w489 -> [w506 _]
                      disable-tunnel: w488 -> [w501 _]
                      disable-tunnel: w487 -> [w499 _]
                      disable-tunnel: w486 -> [w498 _]
                      disable-tunnel: w474 -> [w497 _]
                      disable-tunnel: w485 -> [_ w535]
                      disable-tunnel: w484 -> [_ w534]
                      disable-tunnel: w483 -> [_ w533]
                      disable-tunnel: [_ w532] -> w482
                      disable-tunnel: [_ w531] -> w481
                      disable-tunnel: [_ w530] -> w480
                      disable-tunnel: w479 -> [w496 _]
                      disable-tunnel: w476 -> [w491 w529]
                      disable-tunnel: w478 -> [w494 _]
                      disable-tunnel: w477 -> [w490 _]
                      frame Disabled {
                        # "WARNING!\nUpgrade this code to generate AVI video files instead of individual images.\nUse the code in the \"AVI U16 write-read multi frame.vi\" in C:\\UCL\\RIG 3\\Source Code\\Prototyping\\AVI saves prototyping."
                        n114 = case shown="True" w496 {
                          tunnel: w491 -> [w508 w509]
                          tunnel: [w507 w509] -> w495
                          frame False {
                            # "Vertical"
                            n115 = Transpose 2D Array(2D array=w508) -> (transposed array=w507:refnum<k34>[][])
                          }
                          frame True {
                            # "Horisontal"
                          }
                        }
                        n116 = call "AVI Video Save.vi"("Image Pixels"=w491) -> ()  [unwired: 9 in, 2 out]
                        n117 = call "IMAQ ArrayToImage"("Image Pixels (I16)"=w495, "Image"=w506) -> ("error out"=w502:errorcluster, "Image Out"=w505:T12)  [unwired: 8 in]
                        n118 = Concatenate Strings(w494, "1" ("string")) -> (w492:string)
                        n119 = call "Generate volume image path.vi"("Channel to process"=w490, "Volume index"=w499, "Number of planes"=w498, "Plane index (within its volume)"=w497, "Folder path"=w501) -> ("File path"=w500:path)  [unwired: 5 in, 1 out]
                        n120 = disable-structure shown="Enabled" {
                          disable-tunnel: w497 -> [w520 _]
                          disable-tunnel: w505 -> [w519 w528]
                          disable-tunnel: [w518 w528] -> w504
                          disable-tunnel: [w516 w527] -> w503
                          disable-tunnel: w502 -> [w517 w527]
                          disable-tunnel: w492 -> [w515 _]
                          frame Enabled {
                            w522 = T11 1 items=["Grayscale (U8)", "Grayscale (I16)", "Grayscale (SGL)", "Complex (CSG)", "RGB (U32)", "HSL (U32)", "RGB (U64)"] ("Image Type")
                            # "Warning!\n-32767 or -32768??"
                            n121 = Number To Decimal String(number=w520) -> (decimal integer string=w523:string)  [unwired: 1 in]
                            n122 = Concatenate Strings(w515, w523) -> (w524:string)
                            n123 = call "IMAQ Create"("Image Name"=w524, "Image Type"=w522, "error in (no error)"=w517) -> ("New Image"=w525:T12, "error out"=w526:errorcluster)  [unwired: 2 in]
                            n124 = call "IMAQ Add"("Image Src A"=w519, "Constant"=i16 -32768, "Image Dst"=w525, "error in (no error)"=w526) -> ("Image Dst Out"=w518:T12, "error out"=w516:errorcluster)  [unwired: 3 in]
                          }
                          frame Disabled {
                          }
                        }
                        n125 = disable-structure shown="Enabled" {
                          disable-tunnel: w504 -> [w512 _]
                          disable-tunnel: w503 -> [w511 _]
                          disable-tunnel: w500 -> [w510 _]
                          frame Enabled {
                            n126 = call-poly "IMAQ Write File 2"("error in (no error)"=w511, "File Path"=w510, "Image"=w512) -> ("error out"=w514:errorcluster, "Image Out (duplicate)"=w513:T12)  [unwired: 7 in]
                            n127 = call "IMAQ Dispose"("Image"=w513, "error in (no error)"=w514) -> ()  [unwired: 4 in, 1 out]
                          }
                          frame Disabled {
                          }
                        }
                      }
                      frame Enabled {
                        # "WARNING!\nPotential issues with this basic implementation can be as follows:\n\n1. It uses the AVI2 implementation which doesn't support generating videos >2GB. \nThe logic would need to be upgraded similarly to the timelapse imaging code to split the recording into multiple AVI files of <2GB and named suitable.\n\n2. It will place all recorded images in the same AVI file even when they belong to different ROIs like different volumes or different squares.\n\n3. It may error out when ROI sizes differ. To be tested.\nNote to revert to the previous functionality generating individual images simply enable the disabled cases of the 3 yellow structures."
                        n128 = To Unsigned Long Integer(number=w529) -> (unsigned 32bit integer=w537:u32)
                        n129 = call "IMAQ ArrayToColorImage"("Image Pixels (U32)"=w537, "Image"=w534, "error in (no error)"=w533) -> ("Image Out"=w538:T12, "error out"=w536:errorcluster)  [unwired: 1 in, 1 out]
                        n130 = call "IMAQ AVI2 Write Frame"("error in (no error)"=w536, "Image"=w538, "AVI Refnum"=w535) -> ("error out"=w532:errorcluster, "Image Out (duplicate)"=w530:T12, "AVI Refnum (duplicate)"=w531:T13)  [unwired: 6 in]
                      }
                    }
                  }
                }
                n131 = disable-structure "Diagram Disable Structure" shown="Enabled" {
                  disable-tunnel: w444 -> [w458 _]
                  disable-tunnel: w447 -> [w457 _]
                  disable-tunnel: w445 -> [w456 _]
                  frame Enabled {
                    n132 = call "IMAQ AVI2 Close"("error in (no error)"=w457, "AVI Refnum"=w458) -> ()  [unwired: 9 in, 1 out]
                    n133 = call "IMAQ Dispose"("Image"=w456) -> ()  [unwired: 5 in, 1 out]
                  }
                  frame Disabled {
                  }
                }
                n134 = call "IMAQ Dispose"("Image"=w446, "error in (no error)"=w447) -> ("error out"=w434:errorcluster)  [unwired: 4 in]
                n135 = flat-sequence {
                  tunnel: w434 -> [w449]
                  tunnel: [w449] -> w433
                  frame #0 {
                    n136 = Request Deallocation(TRUE ("flag")) -> ()
                  }
                }
              }
              frame Error {
              }
            }
          }
        }
      }
    }
    frame True {
    }
  }
  "error out" <- w14
  "tdms file out" <- w1
